vi "Set LPF State.vi"(8 "error in (no error)":errorcluster, 10 "LPF State":T1, 11 "Instrument.1820 in":refnum<class "Instrument.Oxford1820.lvclass">) -> (0 "error out":errorcluster, 2 "Response":string, 3 "Instrument.1820 in":refnum<class "Instrument.Oxford1820.lvclass">)   [LabVIEW 2019, in "Instrument.Oxford1820.lvclass"]
uses:
  Instrument.Oxford1820.lvclass
  C:/Program Files (x86)/National Instruments/LabVIEW 2019/user.lib/LevyLab/Instrument Framework/Instrument/Instrument.lvclass
  <instrlib>/Mercury iXX/Public/Libraries/Magnet/Controls/Switch Heater.ctl
  Typedefs/Instrument.Oxford1820.Commands-enum.ctl
  8d3ba4c3-ebb5-4e76-9bed-50ee4c949ff9.vi
  8d3ba4c3-ebb5-4e76-9bed-50ee4c949ff9.vi/0c45259a-164b-47bc-93fe-0b9bc08f2608.vi
  8d3ba4c3-ebb5-4e76-9bed-50ee4c949ff9.vi/0c45259a-164b-47bc-93fe-0b9bc08f2608.vi/8c7bf6fa-4352-4c3f-9a35-102f53b6835d.vi
  8d3ba4c3-ebb5-4e76-9bed-50ee4c949ff9.vi/0c45259a-164b-47bc-93fe-0b9bc08f2608.vi/009656b0-2360-4b2e-bb91-d8cd65c16dff.vi
  <userlib>/LevyLab/Instrument Framework/Instrument/API/RemoteClient.vi
  <vilib>/Utility/Data Type/Get Type Information.vi
  <vilib>/JDP Science/JSONtext/JSON text to Variant.vi
  <vilib>/JDP Science/JSONtext/LVClass Serializer/JSONtext LVClass Serializer.lvclass
  <instrlib>/Mercury iXX/Public/Libraries/Magnet.lvlib
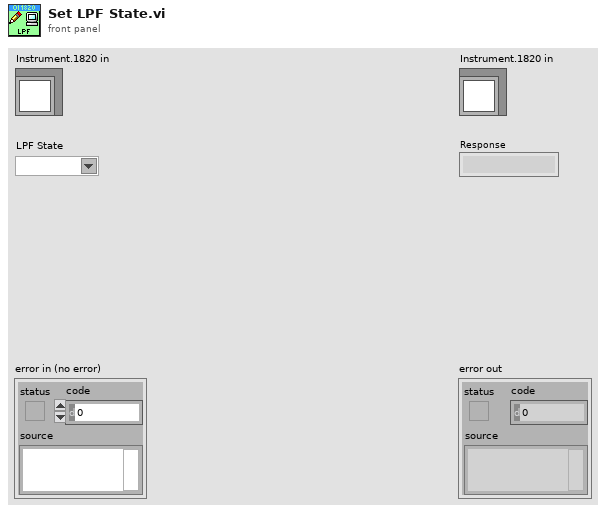
[diagram p1: front panel]
types:
  T1 = typedef "Mercury iXX.lvlib/Magnet.lvlib/Switch Heater.ctl" = string
  T2 = typedef "Instrument.Oxford1820.lvclass/Instrument.Oxford1820.Commands-enum.ctl" = enum16{"setAction", "setTarget", "setSwitchHeat", "setLambda", "setFillMode", "setNeedleValve", "setMagnetField", "getStatus", "getTarget", "getSwitchHeat", "getPSUField", "setSequenceStatus", "getMagnetField"}
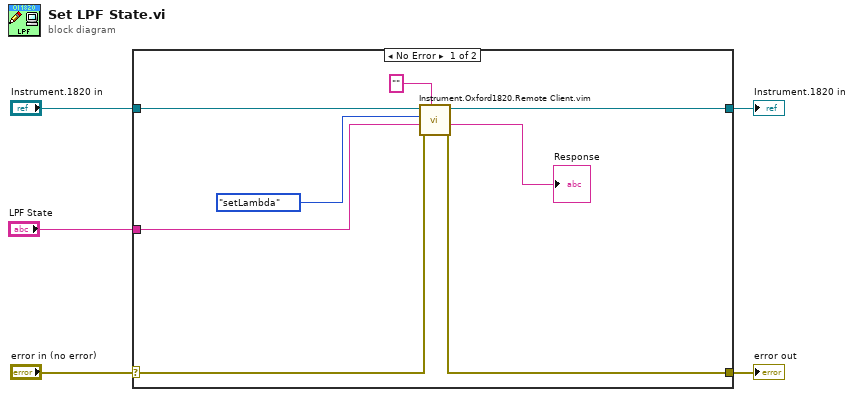
[diagram p0: block diagram]
diagram:
  n1 = case shown="No Error" "error in (no error)" {
    selector: "error in (no error)" -> [w13 w15]
    tunnel: [w8 w15] -> w4
    tunnel: [w7 w14] -> w2
    tunnel: "Instrument.1820 in" -> [w10 w14]
    tunnel: "LPF State" -> [w12 _]
    frame No Error {
      n2 = call "Instrument.Oxford1820.Remote Client.vim"("Data Out type"="", "error in (no error)"=w13, "Data"=w12, "Commands"=Instrument.Oxford1820.Commands-enum."setLambda", "Instrument.1820 in"=w10) -> ("error out"=w8:errorcluster, "Data out"=→"Response":string, "Instrument.1820 out"=w7:refnum<class "Instrument.Oxford1820.lvclass">)  [unwired: 4 in]
    }
    frame Error {
    }
  }
  "error out" <- w4
  "Instrument.1820 in" <- w2
